vi "Read Optimization Results.vi"(7 "Bus by ID Array":T1[](array[typedef]), 8 "error in":errorcluster, 11 "Generic Optimization in":refnum<class "Generic Optimization.lvclass">) -> (0 "error out":errorcluster, 2 "Solution Result":string="Optimal", 3 "Generic Optimization out":refnum<class "Generic Optimization.lvclass">)   [LabVIEW 2018, in "Generic Optimization Actor.lvlib" / "Generic Optimization.lvclass"]
uses:
  Generic Optimization.lvclass
  C:/Users/Administrator/Desktop/2018LabVIEW EMS/EMS Generic Actor/EMS Generic/EMS Generic.lvclass
  C:/Users/Administrator/Desktop/2018LabVIEW EMS/Device Communication and Control Abstract Actor/Device Communication and Control Abstract/Device Communication and Control Abstract.lvclass
  Optimization Controls/Bus by ID.ctl
  <vilib>/ORNL/CSEISMIC DDS/CSEISMIC DDS Base/Data Types/Controls/DeviceID.ctl
  <vilib>/ORNL/CSEISMIC DDS/CSEISMIC DDS Base/Data Types/DER_SetPointV.ctl
  <vilib>/ORNL/CSEISMIC DDS/CSEISMIC DDS Base/Data Types/DER_SetPointF.ctl
  Generic Optimization.lvclass/Generic Optimization.ctl
  <vilib>/ORNL/CSEISMIC DDS/CSEISMIC DDS Base/Data Types/Controls/DeviceClass Selector.ctl
  <vilib>/ORNL/CSEISMIC DDS/CSEISMIC DDS Base/Data Types/DER_SetPointQ.ctl
  <vilib>/ORNL/CSEISMIC DDS/CSEISMIC DDS Base/Data Types/DER_SetPointP.ctl
  <vilib>/ActorFramework/Actor/Actor.lvclass/Actor.ctl
  Device Communication and Control Abstract Actor/Device Communication and Control Abstract/Device Communication and Control Abstract.lvclass/Device Communication and Control Abstract.ctl
  Device Communication and Control Abstract Actor/Device Communication and Control Abstract Messages/Set DER SetPointQ Msg/Set DER SetPointQ Msg.lvclass/Set DER SetPointQ Msg.ctl
  <vilib>/ActorFramework/Message Enqueuer/Message Enqueuer.lvclass/Message Enqueuer.ctl
  Device Communication and Control Abstract Actor/Device Communication and Control Abstract Messages/Set DER SetPointP Msg/Set DER SetPointP Msg.lvclass/Set DER SetPointP Msg.ctl
  Device Communication and Control Abstract Actor/Device Communication and Control Abstract Messages/Set DER SetPointV Msg/Set DER SetPointV Msg.lvclass/Set DER SetPointV Msg.ctl
  Device Communication and Control Abstract Actor/Device Communication and Control Abstract Messages/Set DER SetPointF Msg/Set DER SetPointF Msg.lvclass/Set DER SetPointF Msg.ctl
  <vilib>/ORNL/CSEISMIC DDS/CSEISMIC DDS Base/Data Types/ForecastData_Data.ctl
  Device Communication and Control Abstract Actor/Device Communication and Control Abstract Messages/Set ForecastData Long Msg/Set ForecastData Long Msg.lvclass/Set ForecastData Long Msg.ctl
  <vilib>/ActorFramework/Actor/Read Caller Enqueuer.vi
  Device Communication and Control Abstract Actor/Device Communication and Control Abstract Messages/Set DER SetPointV Msg/Send Set DER SetPointV.vi
  Device Communication and Control Abstract Actor/Device Communication and Control Abstract Messages/Set DER SetPointF Msg/Send Set DER SetPointF.vi
  Device Communication and Control Abstract Actor/Device Communication and Control Abstract Messages/Set DER SetPointQ Msg/Send Set DER SetPointQ.vi
  Device Communication and Control Abstract Actor/Device Communication and Control Abstract Messages/Set DER SetPointP Msg/Send Set DER SetPointP.vi
  Device Communication and Control Abstract Actor/Device Communication and Control Abstract Messages/Set ForecastData Long Msg/Send Set ForecastData Long.vi
  <vilib>/ActorFramework/Message Enqueuer/Enqueue.vi
  Device Communication and Control Abstract Actor/Device Communication and Control Abstract/Device Communication and Control Abstract.lvclass
  C:/Program Files (x86)/National Instruments/LabVIEW 2018/vi.lib/ActorFramework/Actor/Actor.lvclass
  Device Communication and Control Abstract Actor/Device Communication and Control Abstract Messages/Set DER SetPointV Msg/Set DER SetPointV Msg.lvclass
  C:/Program Files (x86)/National Instruments/LabVIEW 2018/vi.lib/ActorFramework/Message/Message.lvclass
  Device Communication and Control Abstract Actor/Device Communication and Control Abstract Messages/Set DER SetPointF Msg/Set DER SetPointF Msg.lvclass
  Device Communication and Control Abstract Actor/Device Communication and Control Abstract Messages/Set DER SetPointQ Msg/Set DER SetPointQ Msg.lvclass
  Device Communication and Control Abstract Actor/Device Communication and Control Abstract Messages/Set DER SetPointP Msg/Set DER SetPointP Msg.lvclass
  Device Communication and Control Abstract Actor/Device Communication and Control Abstract Messages/Set ForecastData Long Msg/Set ForecastData Long Msg.lvclass
  <vilib>/ActorFramework/Message Priority Queue/Priority Enqueue.vi
  <vilib>/ORNL/CSEISMIC DDS/CSEISMIC DDS Base/CSEISMIC DDS.lvclass
  EMS Generic Actor/EMS Generic/EMS Generic.lvclass
panel:
  out "SOC":dbl[][](array[numeric])
  out "PV Power":dbl[][](array[numeric])=[[5.0], [25.0], [25.0], [25.0], [5.0]]
  out "Bus_Voltages":dbl[][](array[numeric])=[[-35.0, -50.0], [-35.0, -50.0], [-35.0, -50.0], [-35.0, -50.0], [-35.0, -50.0]]
  out "GEN_VF":dbl[](array[numeric])
  out "ES_VF":dbl[](array[numeric])=[0.0, 1.0]
  out "QCC":dbl[](array[numeric])
  out "PCC":dbl[](array[numeric])=[10.0, 40.0, 40.0, -10.0, -40.0]
  out "Generator_Reactive":dbl[][](array[numeric])
  out "Generator_Real":dbl[][](array[numeric])=[[5.0], [25.0], [25.0], [25.0], [5.0]]
  out "ES_Reactive":dbl[][](array[numeric])=[[5.0, 0.0], [5.0, 0.0], [5.0, 0.0], [5.0, 0.0], [5.0, 0.0]]
  out "ES_Real":dbl[][](array[numeric])=[[-35.0, -50.0], [-35.0, -50.0], [-35.0, -50.0], [-35.0, -50.0], [-35.0, -50.0]]
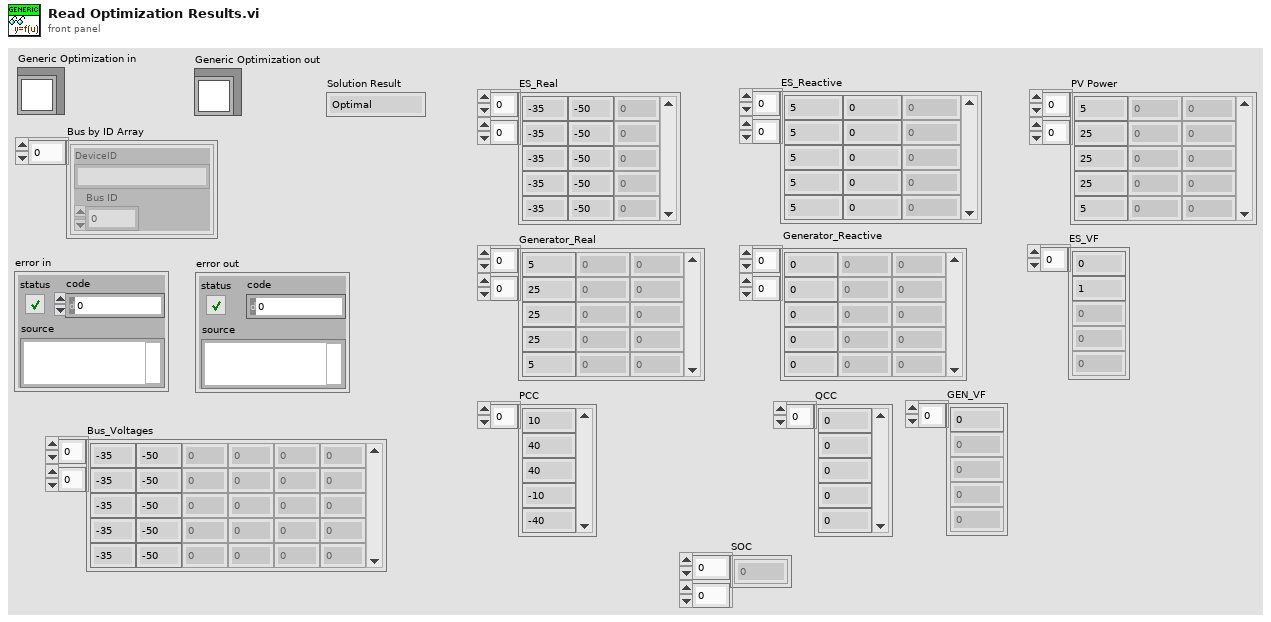
[diagram p1: front panel]
types:
  T1 = typedef "Generic Optimization Actor.lvlib/Generic Optimization.lvclass/Bus by ID.ctl" = cluster{"DeviceID":T2, "Bus ID":dbl}
  T2 = typedef "CSEISMIC DDS.lvlib/CSEISMIC DDS.lvclass/DeviceID.ctl" = string
  T3 = typedef "CSEISMIC DDS.lvlib/CSEISMIC DDS.lvclass/DER_SetPointF.ctl" = cluster{"DeviceID":T2, "Frequency (Hz)":dbl}
  T4 = typedef "CSEISMIC DDS.lvlib/CSEISMIC DDS.lvclass/DER_SetPointV.ctl" = cluster{"DeviceID":T2, "Voltage (V)":dbl}
  T5 = typedef "CSEISMIC DDS.lvlib/CSEISMIC DDS.lvclass/DeviceClass Selector.ctl" = u16
  T6 = typedef "CSEISMIC DDS.lvlib/CSEISMIC DDS.lvclass/ForecastData_Data.ctl" = cluster{"DeviceID":T2, "TargetID":T2, "t0":dbl, "dt":dbl, "Magnitude":dbl[]}
  T7 = typedef "CSEISMIC DDS.lvlib/CSEISMIC DDS.lvclass/DER_SetPointP.ctl" = cluster{"DeviceID":T2, "RealPower (kW)":dbl[]}
  T8 = typedef "CSEISMIC DDS.lvlib/CSEISMIC DDS.lvclass/DER_SetPointQ.ctl" = cluster{"DeviceID":T2, "ReactivePower (kVAR)":dbl[]}
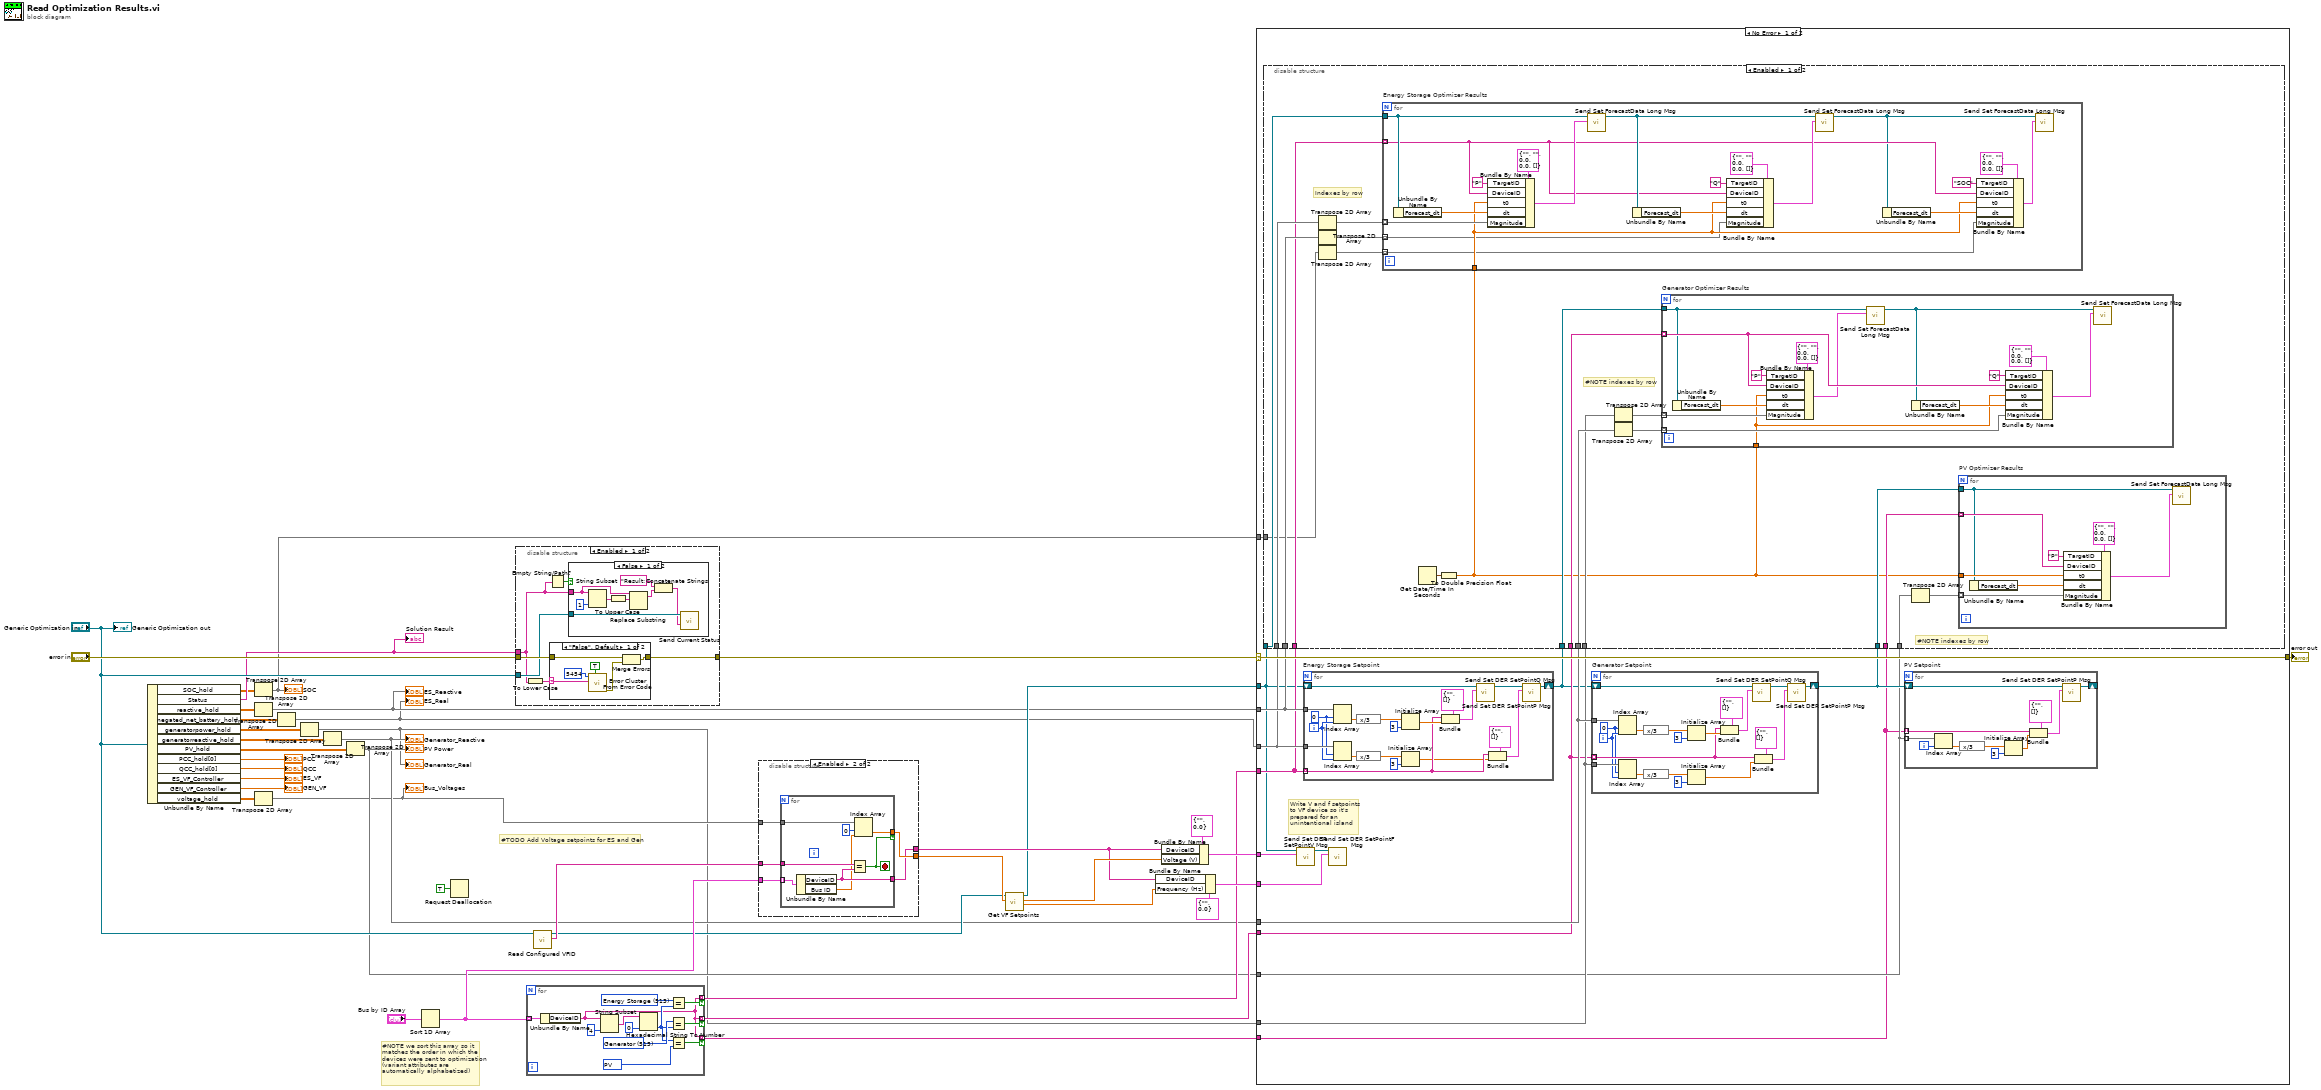
[diagram p0: block diagram]
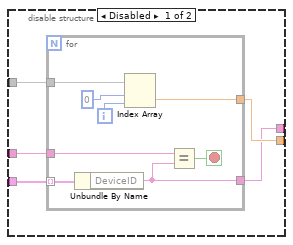
[diagram p2: hidden frame]
diagram:
  # "#NOTE we sort this array so it matches the order in which the devices were sent to optimization (variant attributes are automatically alphabetized)"
  # "#TODO Add Voltage setpoints for ES and Gen"
  n1 = Unbundle By Name("Generic Optimization in") -> ("SOC_hold"=w2:dbl[][], "Status"=w3:string, "reactive_hold"=w19:dbl[][], "negated_net_battery_hold"=w18:dbl[][], "generatorpower_hold"=w17:dbl[][], "generatorreactive_hold"=w16:dbl[][], "PV_hold"=w15:dbl[][], "PCC_hold[0]"=→"PCC":dbl[], "QCC_hold[0]"=→"QCC":dbl[], "ES_VF_Controller"=→"ES_VF":dbl[], "GEN_VF_Controller"=→"GEN_VF":dbl[], "voltage_hold"=w14:dbl[][])
  "Solution Result" <- w3
  n2 = Transpose 2D Array(2D array=w2) -> (transposed array=w1:dbl[][])
  "SOC" <- w1
  n3 = Transpose 2D Array(2D array=w19) -> (transposed array=w7:dbl[][])
  "ES_Reactive" <- w7
  n4 = Transpose 2D Array(2D array=w14) -> (transposed array=w5:dbl[][])
  "Bus_Voltages" <- w5
  n5 = Transpose 2D Array(2D array=w18) -> (transposed array=w6:dbl[][])
  "ES_Real" <- w6
  n6 = Transpose 2D Array(2D array=w17) -> (transposed array=w4:dbl[][])
  "Generator_Real" <- w4
  n7 = Transpose 2D Array(2D array=w16) -> (transposed array=w8:dbl[][])
  "Generator_Reactive" <- w8
  n8 = Transpose 2D Array(2D array=w15) -> (transposed array=w13:dbl[][])
  "PV Power" <- w13
  n9 = Sort 1D Array(array="Bus by ID Array") -> (sorted array=w26:T1[])
  n10 = Request Deallocation(TRUE ("flag")) -> ()
  n11 = disable-structure shown="Enabled" {
    disable-tunnel: "error in" -> [w46 w62]
    disable-tunnel: w3 -> [w41 _]
    disable-tunnel: [w45 w62] -> w36
    disable-tunnel: "Generic Optimization in" -> [w43 _]
    frame Enabled {
      n12 = To Lower Case(string=w41) -> (all lower case string=w44:string)
      n13 = Empty String/Path?(string/path=w41) -> (empty?=w42:bool)
      n14 = case shown="\"False\", Default" w44 {
        selector: w44 -> [w57 _]
        tunnel: w46 -> [w55 w61]
        tunnel: [w56 w61] -> w45
        frame "False", Default {
          n15 = call <vilib>:"Error Cluster From Error Code.vi"("show call chain? (False)"=TRUE, "error message (\"\")"=w57, "error code (0)"=5454) -> ("error out"=w60:errorcluster)  [unwired: 6 in]
          n16 = Merge Errors(w55, w60) -> (w56:errorcluster)
        }
        frame "optimal" {
        }
      }
      n17 = case shown="False" w42 {
        tunnel: w43 -> [w54 _]
        tunnel: w41 -> [w47 _]
        frame False {
          n18 = String Subset(string=w47, length (rest)=1 ("length (rest)")) -> (substring=w51:string)  [unwired: 1 in]
          n19 = To Upper Case(1:w51) -> (0:w52:string)
          n20 = Replace Substring(4:w52, 5:w47) -> (1:w49:string)  [unwired: 2 in, 1 out]
          n21 = Concatenate Strings("Result: " ("string"), w49) -> (w48:string)
          n22 = call "Send Current Status.vi"("Current Status"=w48, "Device Communication and Control Abstract in"=w54) -> ()  [unwired: 8 in, 2 out]
        }
        frame True {
        }
      }
    }
    frame Disabled {
    }
  }
  n23 = for {
    tunnel: w26 -> [w74] mode=indexing
    tunnel: [w64] -> w27 mode=indexing if=w68
    tunnel: [w64] -> w29 mode=indexing if=w67
    tunnel: [w64] -> w28 mode=indexing if=w63
    w65 = T5 514 items=["Invalid"=0, "IED"=256, "DER"=512, "Relay"=768, "Meter"=1024, "Load"=1280, "Forecast"=1536, "Price"=1792, "Energy Storage"=513, "PV"=514, "Generator"=515, "Smart Relay"=769, "PCC"=770, "Smart Meter"=1025, "PMU"=1026, "HVAC"=1281] ("DeviceClass")
    w69 = T5 513 items=["Invalid"=0, "IED"=256, "DER"=512, "Relay"=768, "Meter"=1024, "Load"=1280, "Forecast"=1536, "Price"=1792, "Energy Storage"=513, "PV"=514, "Generator"=515, "Smart Relay"=769, "PCC"=770, "Smart Meter"=1025, "PMU"=1026, "HVAC"=1281] ("DeviceClass")
    w70 = T5 515 items=["Invalid"=0, "IED"=256, "DER"=512, "Relay"=768, "Meter"=1024, "Load"=1280, "Forecast"=1536, "Price"=1792, "Energy Storage"=513, "PV"=514, "Generator"=515, "Smart Relay"=769, "PCC"=770, "Smart Meter"=1025, "PMU"=1026, "HVAC"=1281] ("DeviceClass")
    n24 = Unbundle By Name(w74) -> ("DeviceID"=w64:T2)
    n25 = String Subset(string=w64, length (rest)=4 ("length (rest)")) -> (substring=w72:T2)  [unwired: 1 in]
    n26 = Hexadecimal String To Number(string=w72, default (0uL)=u16 0 ("default (0 U32)")) -> (number=w66:u16)  [unwired: 1 in, 1 out]
    n27 = Equal?(x=w69, y=w66) -> (x = y?=w67:bool)
    n28 = Equal?(x=w70, y=w66) -> (x = y?=w68:bool)
    n29 = Equal?(x=w66, y=w65) -> (x = y?=w63:bool)
  }
  n30 = call "Read Configured VFID.vi"("EMS Generic in"="Generic Optimization in") -> ("VFID"=w25:T2, "EMS Generic out"=w23:refnum<class "Generic Optimization.lvclass">)  [unwired: 8 in, 1 out]
  n31 = disable-structure shown="Enabled" {
    disable-tunnel: w26 -> [w79 w92]
    disable-tunnel: w25 -> [w78 w91]
    disable-tunnel: w5 -> [w77 w90]
    disable-tunnel: [w76 w89] -> w34
    disable-tunnel: [w75 w88] -> w31
    frame Disabled {
      n32 = for {
        tunnel: w79 -> [w87] mode=indexing
        tunnel: w78 -> [w86]
        tunnel: w77 -> [w84]
        tunnel: [w83] -> w76
        tunnel: [w82] -> w75
        i -> [w80]
        stop <- w85 stop-if-true
        n33 = Unbundle By Name(w87) -> ("DeviceID"=w82:T2)
        n34 = Index Array(array=w84, index (row)=0 ("disabled index (row)"), index (col)=w80) -> (element=w83:dbl)
        n35 = Equal?(x=w86, y=w82) -> (x = y?=w85:bool)
      }
    }
    frame Enabled {
      n36 = for {
        tunnel: w92 -> [w100] mode=indexing
        tunnel: w91 -> [w99]
        tunnel: w90 -> [w97]
        tunnel: [w94] -> w89 if=w93
        tunnel: [w98] -> w88
        stop <- w93 stop-if-true
        n37 = Unbundle By Name(w100) -> ("DeviceID"=w98:T2, "Bus ID"=w95:dbl)
        n38 = Equal?(x=w99, y=w98) -> (x = y?=w93:bool)
        n39 = Index Array(array=w97, index (row)=0, index (col)=w95) -> (element=w94:dbl)
      }
    }
  }
  n40 = call-dynamic "Get VF Setpoints.vi"("Per-Unitized VF Voltage Setpoint"=w34, "Generic Optimization in"=w23) -> ("VF Frequency Setpoint"=w24:dbl, "VF Voltage Setpoint"=w33:dbl, "Generic Optimization out"=w22:refnum<class "Generic Optimization.lvclass">)  [unwired: 7 in]
  n41 = Bundle By Name(cluster=T3 {"DeviceID"="", "Frequency (Hz)"=0.0} ("DER_SetPointF"), "DeviceID"=w31, "Frequency (Hz)"=w24) -> (w30:T3)
  n42 = Bundle By Name(cluster=T4 {"DeviceID"="", "Voltage (V)"=0.0} ("DER_SetPointVF"), "DeviceID"=w31, "Voltage (V)"=w33) -> (w35:T4)
  n43 = case shown="No Error" w36 {
    selector: w36 -> [w116 w230]
    tunnel: w27 -> [w108 _]
    tunnel: w4 -> [w110 _]
    tunnel: w8 -> [w111 _]
    tunnel: w22 -> [w109 _]
    tunnel: w29 -> [w112 _]
    tunnel: w7 -> [w114 _]
    tunnel: w6 -> [w113 _]
    tunnel: [w116 w230] -> w39
    tunnel: w35 -> [w102 _]
    tunnel: w13 -> [w105 _]
    tunnel: w28 -> [w104 _]
    tunnel: w30 -> [w103 _]
    tunnel: w1 -> [w101 _]
    frame No Error {
      # "Write V and f setpoints to VF device so it's prepared for an unintentional island"
      n44 = call "Send Set DER SetPointV Msg.vi"("DER_SetPointV"=w102, "SCADA Sub Abstract in"=w109) -> ("dup SCADA Sub Abstract"=w115:refnum<class "Generic Optimization.lvclass">)  [unwired: 8 in, 1 out]
      n45 = for "Energy Storage Setpoint" {
        tunnel: w112 -> [w195] mode=indexing
        tunnel: w113 -> [w205]
        tunnel: w114 -> [w206]
        shift-right: [w208] -> w107
        shift-left: w109 -> [w197]
        i -> [w193]
        w192 = 0 ("disabled index (row)")
        n46 = Index Array(array=w206, index (row)=w192, index (col)=w193) -> (element=w203:dbl)
        n47 = Index Array(array=w205, index (row)=w192, index (col)=w193) -> (element=w204:dbl)
        n48 = expression code="x/3"(w203) -> (w199:dbl)
        n49 = expression code="x/3"(w204) -> (w202:dbl)
        n50 = Initialize Array(w199, 3 ("dimension size")) -> (w198:dbl[])
        n51 = Initialize Array(w202, 3 ("dimension size")) -> (w194:dbl[])
        n52 = Bundle(cluster=T8 {"DeviceID"="", "ReactivePower (kVAR)"=[]} ("DER_SetPointQ"), "DeviceID"=w195, "ReactivePower (kVAR)"=w198) -> (w190:T8)
        n53 = call "Send Set DER SetPointQ Msg.vi"("DER_SetPointQ"=w190, "SCADA Sub Abstract in"=w197) -> ("dup SCADA Sub Abstract"=w209:refnum<class "Generic Optimization.lvclass">)  [unwired: 8 in, 1 out]
        n54 = Bundle(cluster=T7 {"DeviceID"="", "RealPower (kW)"=[]} ("DER_SetPointP"), "DeviceID"=w195, "RealPower (kW)"=w194) -> (w191:T7)
        n55 = call "Send Set DER SetPointP Msg.vi"("DER_SetPointP"=w191, "SCADA Sub Abstract in"=w209) -> ("SCADA Sub Abstract out"=w208:refnum<class "Generic Optimization.lvclass">)  [unwired: 8 in, 1 out]
      }
      n56 = call "Send Set DER SetPointF Msg.vi"("DER_SetPointF"=w103, "SCADA Sub Abstract in"=w115) -> ()  [unwired: 8 in, 2 out]
      n57 = for "Generator Setpoint" {
        tunnel: w108 -> [w215] mode=indexing
        tunnel: w110 -> [w225]
        tunnel: w111 -> [w226]
        shift-right: [w228] -> w106
        shift-left: w107 -> [w217]
        i -> [w213]
        w212 = 0 ("disabled index (row)")
        n58 = Index Array(array=w226, index (row)=w212, index (col)=w213) -> (element=w223:dbl)
        n59 = Index Array(array=w225, index (row)=w212, index (col)=w213) -> (element=w224:dbl)
        n60 = expression code="x/3"(w223) -> (w219:dbl)
        n61 = expression code="x/3"(w224) -> (w222:dbl)
        n62 = Initialize Array(w219, 3 ("dimension size")) -> (w218:dbl[])
        n63 = Initialize Array(w222, 3 ("dimension size")) -> (w214:dbl[])
        n64 = Bundle(cluster=T8 {"DeviceID"="", "ReactivePower (kVAR)"=[]} ("DER_SetPointQ"), "DeviceID"=w215, "ReactivePower (kVAR)"=w218) -> (w210:T8)
        n65 = call "Send Set DER SetPointQ Msg.vi"("DER_SetPointQ"=w210, "SCADA Sub Abstract in"=w217) -> ("dup SCADA Sub Abstract"=w229:refnum<class "Generic Optimization.lvclass">)  [unwired: 8 in, 1 out]
        n66 = Bundle(cluster=T7 {"DeviceID"="", "RealPower (kW)"=[]} ("DER_SetPointP"), "DeviceID"=w215, "RealPower (kW)"=w214) -> (w211:T7)
        n67 = call "Send Set DER SetPointP Msg.vi"("DER_SetPointP"=w211, "SCADA Sub Abstract in"=w229) -> ("SCADA Sub Abstract out"=w228:refnum<class "Generic Optimization.lvclass">)  [unwired: 8 in, 1 out]
      }
      n68 = disable-structure shown="Enabled" {
        disable-tunnel: w114 -> [w136 _]
        disable-tunnel: w113 -> [w135 _]
        disable-tunnel: w112 -> [w134 _]
        disable-tunnel: w111 -> [w129 _]
        disable-tunnel: w110 -> [w128 _]
        disable-tunnel: w109 -> [w127 _]
        disable-tunnel: w108 -> [w126 _]
        disable-tunnel: w107 -> [w124 _]
        disable-tunnel: w106 -> [w123 _]
        disable-tunnel: w105 -> [w122 _]
        disable-tunnel: w104 -> [w121 _]
        disable-tunnel: w101 -> [w118 _]
        frame Enabled {
          # "#NOTE indexes by row"
          # "#NOTE indexes by row"
          # "Indexes by row"
          n69 = Transpose 2D Array(2D array=w135) -> (transposed array=w132:dbl[][])
          n70 = Transpose 2D Array(2D array=w136) -> (transposed array=w133:dbl[][])
          n71 = Transpose 2D Array(2D array=w118) -> (transposed array=w117:dbl[][])
          n72 = Get Date/Time In Seconds() -> (seconds since 1Jan1904=w120:timestamp)
          n73 = To Double Precision Float(number=w120) -> (double precision float=w119:dbl)
          n74 = for "Energy Storage Optimizer Results" {
            tunnel: w134 -> [w163] mode=indexing
            tunnel: w132 -> [w177] mode=indexing
            tunnel: w133 -> [w160] mode=indexing
            tunnel: w119 -> [w161]
            tunnel: w127 -> [w171]
            tunnel: w117 -> [w159] mode=indexing
            n75 = Unbundle By Name(w171) -> ("Forecast_dt"=w176:dbl)
            n76 = Bundle By Name(cluster=T6 {"DeviceID"="", "TargetID"="", "t0"=0.0, "dt"=0.0, "Magnitude"=[]} ("ForecastData"), "TargetID"=T2 "P", "DeviceID"=w163, "t0"=w161, "dt"=w176, "Magnitude"=w177) -> (w169:T6)
            n77 = call "Send Set ForecastData Long Msg.vi"("ForecastData"=w169, "SCADA Sub Abstract in"=w171) -> ("dup SCADA Sub Abstract"=w170:refnum<class "Generic Optimization.lvclass">)  [unwired: 8 in, 1 out]
            n78 = Unbundle By Name(w170) -> ("Forecast_dt"=w173:dbl)
            n79 = Bundle By Name(cluster=T6 {"DeviceID"="", "TargetID"="", "t0"=0.0, "dt"=0.0, "Magnitude"=[]} ("ForecastData"), "TargetID"=T2 "Q", "DeviceID"=w163, "t0"=w161, "dt"=w173, "Magnitude"=w160) -> (w168:T6)
            n80 = call "Send Set ForecastData Long Msg.vi"("ForecastData"=w168, "SCADA Sub Abstract in"=w170) -> ("dup SCADA Sub Abstract"=w162:refnum<class "Generic Optimization.lvclass">)  [unwired: 8 in, 1 out]
            n81 = Unbundle By Name(w162) -> ("Forecast_dt"=w165:dbl)
            n82 = Bundle By Name(cluster=T6 {"DeviceID"="", "TargetID"="", "t0"=0.0, "dt"=0.0, "Magnitude"=[]} ("ForecastData"), "TargetID"=T2 "SOC", "DeviceID"=w163, "t0"=w161, "dt"=w165, "Magnitude"=w159) -> (w167:T6)
            n83 = call "Send Set ForecastData Long Msg.vi"("ForecastData"=w167, "SCADA Sub Abstract in"=w162) -> ()  [unwired: 8 in, 2 out]
          }
          n84 = Transpose 2D Array(2D array=w128) -> (transposed array=w131:dbl[][])
          n85 = Transpose 2D Array(2D array=w129) -> (transposed array=w130:dbl[][])
          n86 = for "Generator Optimizer Results" {
            tunnel: w126 -> [w150] mode=indexing
            tunnel: w131 -> [w157] mode=indexing
            tunnel: w130 -> [w151] mode=indexing
            tunnel: w119 -> [w149]
            tunnel: w124 -> [w148]
            n87 = Unbundle By Name(w148) -> ("Forecast_dt"=w156:dbl)
            n88 = Bundle By Name(cluster=T6 {"DeviceID"="", "TargetID"="", "t0"=0.0, "dt"=0.0, "Magnitude"=[]} ("ForecastData"), "TargetID"=T2 "P", "DeviceID"=w150, "t0"=w149, "dt"=w156, "Magnitude"=w157) -> (w145:T6)
            n89 = call "Send Set ForecastData Long Msg.vi"("ForecastData"=w145, "SCADA Sub Abstract in"=w148) -> ("dup SCADA Sub Abstract"=w147:refnum<class "Generic Optimization.lvclass">)  [unwired: 8 in, 1 out]
            n90 = Unbundle By Name(w147) -> ("Forecast_dt"=w153:dbl)
            n91 = Bundle By Name(cluster=T6 {"DeviceID"="", "TargetID"="", "t0"=0.0, "dt"=0.0, "Magnitude"=[]} ("ForecastData"), "TargetID"=T2 "Q", "DeviceID"=w150, "t0"=w149, "dt"=w153, "Magnitude"=w151) -> (w146:T6)
            n92 = call "Send Set ForecastData Long Msg.vi"("ForecastData"=w146, "SCADA Sub Abstract in"=w147) -> ()  [unwired: 8 in, 2 out]
          }
          n93 = Transpose 2D Array(2D array=w122) -> (transposed array=w125:dbl[][])
          n94 = for "PV Optimizer Results" {
            tunnel: w121 -> [w140] mode=indexing
            tunnel: w125 -> [w143] mode=indexing
            tunnel: w119 -> [w139]
            tunnel: w123 -> [w138]
            n95 = Unbundle By Name(w138) -> ("Forecast_dt"=w142:dbl)
            n96 = Bundle By Name(cluster=T6 {"DeviceID"="", "TargetID"="", "t0"=0.0, "dt"=0.0, "Magnitude"=[]} ("ForecastData"), "TargetID"=T2 "P", "DeviceID"=w140, "t0"=w139, "dt"=w142, "Magnitude"=w143) -> (w137:T6)
            n97 = call "Send Set ForecastData Long Msg.vi"("ForecastData"=w137, "SCADA Sub Abstract in"=w138) -> ()  [unwired: 8 in, 2 out]
          }
        }
        frame Disabled {
        }
      }
      n98 = for "PV Setpoint" {
        tunnel: w104 -> [w182] mode=indexing
        tunnel: w105 -> [w188] mode=indexing
        shift-right: [w189] -> _
        shift-left: w106 -> [w184]
        i -> [w180]
        n99 = Index Array(array=w188, index=w180) -> (element=w187:dbl)
        n100 = expression code="x/3"(w187) -> (w186:dbl)
        n101 = Initialize Array(w186, 3 ("dimension size")) -> (w181:dbl[])
        n102 = Bundle(cluster=T7 {"DeviceID"="", "RealPower (kW)"=[]} ("DER_SetPointP"), "DeviceID"=w182, "RealPower (kW)"=w181) -> (w179:T7)
        n103 = call "Send Set DER SetPointP Msg.vi"("DER_SetPointP"=w179, "SCADA Sub Abstract in"=w184) -> ("SCADA Sub Abstract out"=w189:refnum<class "Generic Optimization.lvclass">)  [unwired: 8 in, 1 out]
      }
    }
    frame Error {
    }
  }
  "error out" <- w39
  "Generic Optimization out" <- "Generic Optimization in"
